vi "Read Actual Server Identity.vi"(10 "server errors":string, 11 "client in":refnum<class "OpenSSH Client.lvclass">) -> (2 "fingerprint":string, 3 "client out":refnum<class "OpenSSH Client.lvclass">)   [LabVIEW 2020, in "NI_SSH.lvlib" / "OpenSSH Client.lvclass"]
uses:
  <vilib>/net/SSH/Client/OpenSSH/OpenSSH Client.lvclass
  e:/builds/penguin/labview/branches/2020/dev/dist/vi.lib/net/SSH/Client/Generic/Generic Client.lvclass
  <vilib>/Subprocess/Subprocess/Subprocess.lvclass
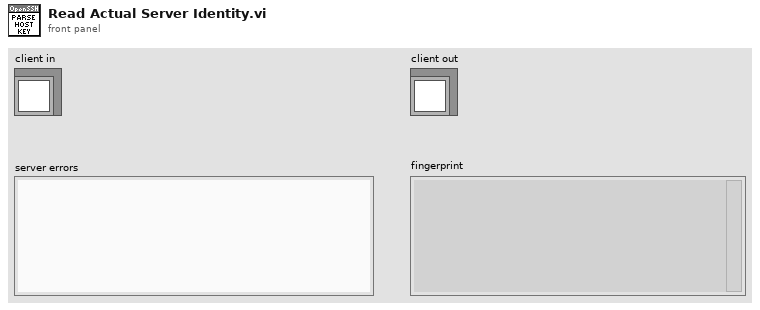
[diagram p1: front panel]
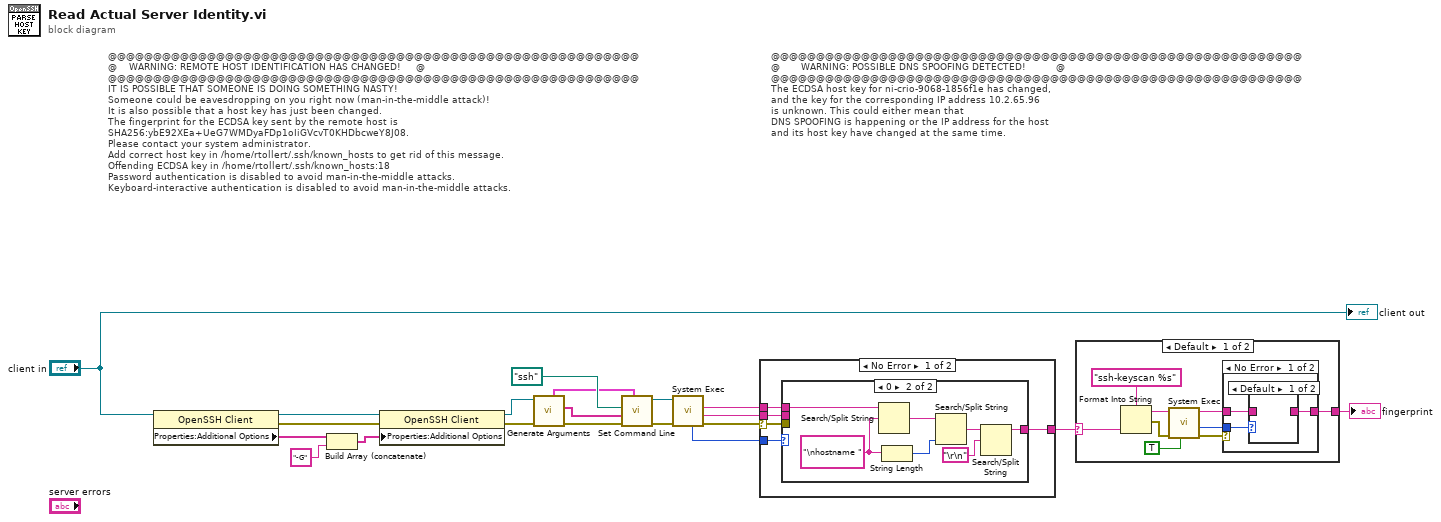
[diagram p0: block diagram]
diagram:
  # "@@@@@@@@@@@@@@@@@@@@@@@@@@@@@@@@@@@@@@@@@@@@@@@@@@@@@@@@@@@\n@       WARNING: POSSIBLE DNS SPOOFING DETECTED!          @\n@@@@@@@@@@@@@@@@@@@@@@@@@@@@@@@@@@@@@@@@@@@@@@@@@@@@@@@@@@@\nThe ECDSA host key for ni-crio-9068-1856f1e has changed,\nand the key for the corresponding IP address 10.2.65.96\nis unknown. This could either mean that\nDNS SPOOFING is happening or the IP address for the host\nand its host key have changed at the same time."
  # "@@@@@@@@@@@@@@@@@@@@@@@@@@@@@@@@@@@@@@@@@@@@@@@@@@@@@@@@@@@\n@    WARNING: REMOTE HOST IDENTIFICATION HAS CHANGED!     @\n@@@@@@@@@@@@@@@@@@@@@@@@@@@@@@@@@@@@@@@@@@@@@@@@@@@@@@@@@@@\nIT IS POSSIBLE THAT SOMEONE IS DOING SOMETHING NASTY!\nSomeone could be eavesdropping on you right now (man-in-the-middle attack)!\nIt is also possible that a host key has just been changed.\nThe fingerprint for the ECDSA key sent by the remote host is\nSHA256:ybE92XEa+UeG7WMDyaFDp1oIiGVcvT0KHDbcweY8J08.\nPlease contact your system administrator.\nAdd correct host key in /home/rtollert/.ssh/known_hosts to get rid of this message.\nOffending ECDSA key in /home/rtollert/.ssh/known_hosts:18\nPassword authentication is disabled to avoid man-in-the-middle attacks.\nKeyboard-interactive authentication is disabled to avoid man-in-the-middle attacks."
  n1 = property on="Property Node" class="OpenSSH Client"(reference="client in") -> (reference out=w9:refnum<class "OpenSSH Client.lvclass">, error out=w11:errorcluster, "Properties:Additional Options"=w13:string[])  [unwired: 1 in]
  n2 = Build Array (concatenate)(w13, "-G") -> (w10:string[])
  n3 = property on="Property Node" class="OpenSSH Client"(reference=w9, error in=w11, "Properties:Additional Options"=w10) -> (reference out=w8:refnum<class "OpenSSH Client.lvclass">, error out=w7:errorcluster)
  n4 = call-dynamic "Generate Arguments.vi"("error in (no error)"=w7, "client in"=w8) -> ("error out"=w4:errorcluster, "arguments"=w5:string[], "environment variables"=w3:cluster{"name":string, "value":string}[])  [unwired: 6 in, 1 out]
  n5 = call <vilib>:"Set Command Line.vi"("environment variables"=w3, "error in (no error)"=w4, "arguments"=w5, "path"=path "ssh") -> ("error out"=w1:errorcluster, "subprocess out"=w2:refnum<class "Subprocess.lvclass">)  [unwired: 6 in]
  n6 = call <vilib>:"System Exec.vi"("error in (no error)"=w1, "subprocess in"=w2) -> ("error out"=w16:errorcluster, "standard error"=w17:string, "standard output"=w18:string, "return code"=w19:i32)  [unwired: 5 in, 1 out]
  n7 = case shown="No Error" w16 {
    selector: w16 -> [w22 _]
    tunnel: w19 -> [w25 _]
    tunnel: w18 -> [w24 _]
    tunnel: w17 -> [w23 _]
    tunnel: [w21 _] -> w15
    frame No Error {
      n8 = case shown="0" w25 {
        tunnel: w24 -> [_ w32]
        tunnel: w23 -> [_ _]
        tunnel: w22 -> [_ _]
        tunnel: [_ w26] -> w21
        frame Default {
        }
        frame 0 {
          w31 = "\nhostname " ("search string/char (-)")
          n9 = Search/Split String(string=w32, search string/char (-)=w31) -> (match + rest of string=w30:string)  [unwired: 1 in, 2 out]
          n10 = String Length(string=w31) -> (length=w29:i32)
          n11 = Search/Split String(string=w30, offset (0)=w29) -> (match + rest of string=w28:string)  [unwired: 1 in, 2 out]
          n12 = Search/Split String(string=w28, search string/char (-)="\r\n" ("End of Line Constant")) -> (substring before match=w26:string)  [unwired: 1 in, 2 out]
        }
      }
    }
    frame Error {
    }
  }
  n13 = case shown="Default" w15 {
    selector: w15 -> [w40 _]
    tunnel: [w33 _] -> w14
    frame Default {
      n14 = Format Into String(format string="ssh-keyscan %s", w40) -> (resulting string=w39:string, error out=w38:errorcluster)  [unwired: 2 in]
      n15 = call <vilib>:"System Exec.vi"("run minimized? (F)"=TRUE, "error in (no error)"=w38, "command line"=w39) -> ("error out"=w37:errorcluster, "return code"=w36:i32, "standard output"=w35:string)  [unwired: 5 in, 1 out]
      n16 = case shown="No Error" w37 {
        tunnel: w36 -> [w44 _]
        tunnel: w35 -> [w43 _]
        tunnel: [w42 _] -> w33
        frame No Error {
          n17 = case shown="Default" w44 {
            tunnel: w43 -> [_ w45]
            tunnel: [_ w45] -> w42
            frame Default {
            }
            frame 0 {
            }
          }
        }
        frame Error {
        }
      }
    }
    frame "" {
    }
  }
  "fingerprint" <- w14
  "client out" <- "client in"
